vi "传感器数据.vi"() -> (2 "PLCchuanganqishuju":T1 {"Factorysensor2" format="%#.3f"; "输出轴移栽位移" format="%#.3f"; "输出轴旋转角度" format="%#.3f"; "Factorysensor" format="%#.3f"; "吸收电流" format="%#.3f"; "输出扭矩(大)" format="%#.3f"; "输出扭矩(小)" format="%#.3f"; "输入扭矩" format="%#.3f"; "输入编码位移" format="%#.3f"; "工装移载位移" format="%#.3f"; "输入移载位移" format="%#.3f"; "输入旋转位移" format="%#.3f"}, 3 "传感器读数":T1 {"Factorysensor2" format="%#.3f"; "输出轴移栽位移" format="%#.3f"; "输出轴旋转角度" format="%#.3f"; "Factorysensor" format="%#.3f"; "吸收电流" format="%#.3f"; "输出扭矩(大)" format="%#.3f"; "输出扭矩(小)" format="%#.3f"; "输入扭矩" format="%#.3f"; "输入编码位移" format="%#.3f"; "工装移载位移" format="%#.3f"; "输入移载位移" format="%#.3f"; "输入旋转位移" format="%#.3f"})   [LabVIEW 2020]
uses:
  Libraries/S7/S7.lvlib
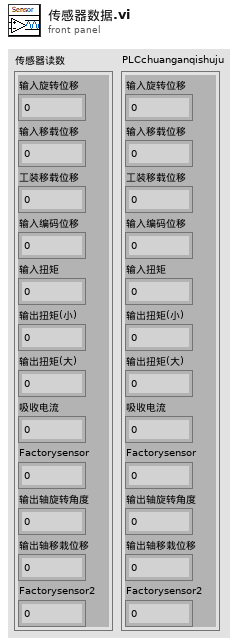
[diagram p1: front panel]
types:
  T1 = cluster{"输入旋转位移":sgl, "输入移载位移":sgl, "工装移载位移":sgl, "输入编码位移":sgl, "输入扭矩":sgl, "输出扭矩(小)":sgl, "输出扭矩(大)":sgl, "吸收电流":sgl, "Factorysensor":sgl, "输出轴旋转角度":sgl, "输出轴移栽位移":sgl, "Factorysensor2":sgl}
  T2 = cluster{"输入轴扭矩":dbl, "输出轴扭矩小量程":dbl, "输出轴扭矩大量程":dbl}
  T3 = typedef "S7.lvlib/Read_Data (Reply Payload)--cluster.ctl" = cluster{"读取成功":bool, "数据":u32[], "Read_Data_error":errorcluster}
  T4 = cluster{sgl, sgl, sgl, sgl, sgl, sgl, sgl, sgl, sgl, sgl, sgl, sgl}
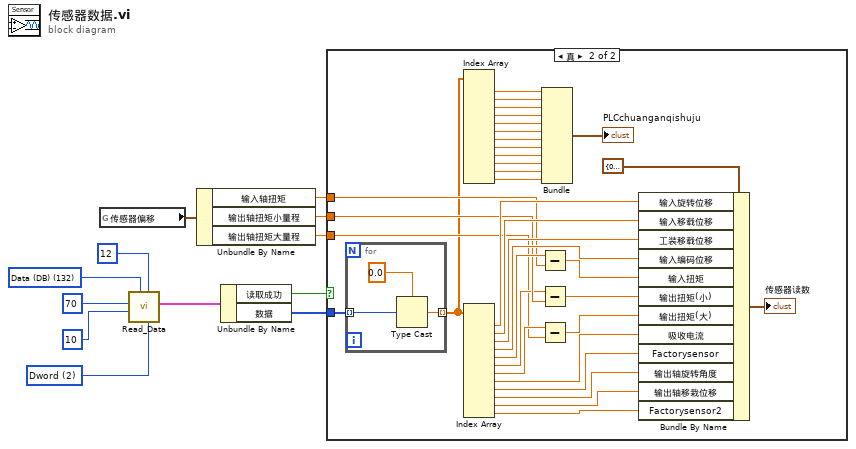
[diagram p0: block diagram]
diagram:
  w9 = u16 2 items=["byte", "word", "Dword"] ("数据类型")
  w10 = u8 132 items=["I/O (P)"=128, "Input (I)"=129, "Output (Q)"=130, "Bit Memory (M)"=131, "Data (DB)"=132, "Instance Data (DI)"=133, "Local Data (L)"=134, "Predecessor Local Data (VL)"=135] ("寄存器类型")
  n1 = global read "传感器偏移.vi" "传感器偏移"() -> (w4:T2)
  n2 = call "Read_Data.vi"("数据类型"=w9, "读取长度"=u16 12, "寄存器类型"=w10, "起始地址"=u32 10, "DB #"=u16 70) -> ("Reply Payload"=w7:T3)  [unwired: 4 in, 2 out]
  n3 = Unbundle By Name(w4) -> ("输入轴扭矩"=w3:dbl, "输出轴扭矩小量程"=w2:dbl, "输出轴扭矩大量程"=w1:dbl)
  n4 = Unbundle By Name(w7) -> ("读取成功"=w5:bool, "数据"=w6:u32[])
  n5 = case shown="真" w5 {
    tunnel: w6 -> [_ w47]
    tunnel: w3 -> [_ w39]
    tunnel: w2 -> [_ w38]
    tunnel: w1 -> [_ w34]
    frame False {
    }
    frame True {
      n6 = for {
        tunnel: w47 -> [w49] mode=indexing
        tunnel: [w48] -> w28 mode=indexing
        n7 = Type Cast(type=sgl 0.0, x=w49) -> (*(type *) &x=w48:sgl)
      }
      n8 = Index Array(array=w28) -> (element #1=w29:sgl, element #2=w27:sgl, element #3=w26:sgl, element #4=w25:sgl, element #5=w24:sgl, element #6=w23:sgl, element #7=w22:sgl, element #8=w21:sgl, element #9=w20:sgl, element #10=w19:sgl, element #11=w18:sgl, element #12=w16:sgl)  [unwired: 12 in]
      n9 = Index Array(array=w28) -> (element #1=w46:sgl, element #2=w45:sgl, element #3=w44:sgl, element #4=w43:sgl, element #5=w42:sgl, element #6=w37:sgl, element #7=w35:sgl, element #8=w41:sgl, element #9=w32:sgl, element #10=w31:sgl, element #11=w30:sgl, element #12=w15:sgl)  [unwired: 12 in]
      n10 = Subtract(x=w42, y=w39) -> (x-y=w40:dbl)
      n11 = Subtract(x=w37, y=w38) -> (x-y=w36:dbl)
      n12 = Subtract(x=w35, y=w34) -> (x-y=w33:dbl)
      n13 = Bundle(w29, w27, w26, w25, w24, w23, w22, w21, w20, w19, w18, w16) -> (→"PLCchuanganqishuju":T4)  [unwired: 1 in]
      n14 = Bundle By Name(cluster=T1 {"输入旋转位移"=0.0, "输入移载位移"=0.0, "工装移载位移"=0.0, "输入编码位移"=0.0, "输入扭矩"=0.0, "输出扭矩(小)"=0.0, "输出扭矩(大)"=0.0, "吸收电流"=0.0, "Factorysensor"=0.0, "输出轴旋转角度"=0.0, "输出轴移栽位移"=0.0, "Factorysensor2"=0.0} ("传感器读数"), "输入旋转位移"=w46, "输入移载位移"=w45, "工装移载位移"=w44, "输入编码位移"=w43, "输入扭矩"=w40, "输出扭矩(小)"=w36, "输出扭矩(大)"=w33, "吸收电流"=w41, "Factorysensor"=w32, "输出轴旋转角度"=w31, "输出轴移栽位移"=w30, "Factorysensor2"=w15) -> (→"传感器读数":T1)
    }
  }
